vi "Check Writer Backpressure.vi"(8 "error in (no error)":errorcluster, 10 "Timeout (ms)":i32, 11 "CIF_CIPC_Chn in":refnum<class "CIF_CIPC_Chn.lvclass">) -> (0 "error out":errorcluster, 2 "timed out?":bool)   [LabVIEW 2021, in "CIF_CIPC_Chn.lvclass"]
uses:
  CIF_CIPC_Chn.lvclass
  D:/dev/Packages/CIF_Channels_Core/src/CIFChannels/CIFChannels.lvclass
  CIFChannels/CIFChannels.lvclass/CIFChannels.ctl
  CIF_CIPC_Chn.lvclass/CIF_CIPC_Chn.ctl
  CIFChannels/Accessors/Read FIFO Backpressure.vi
  080cd5e1-c136-44b9-98fd-184f8e575b7e.vi/3d5c1244-b460-4622-96d1-ee1e369932ac.vi
  <vilib>/CIF Foundation/CIF CIPC/Utilities/Get Size.vi
  080cd5e1-c136-44b9-98fd-184f8e575b7e.vi/b3361ac9-0b85-4d75-8feb-76d028d0c03f.vi
  <vilib>/CIF Foundation/CIF CIPC/SubVIs/Get Element Write Position.vi
  <vilib>/CIF Foundation/CIF CIPC/SubVIs/Wait For N Elements Available.vi
  <vilib>/CIF Foundation/CIF CIPC/SubVIs/Check Error.vi
  <vilib>/CIF Foundation/CIF CIPC/SubVIs/Get dll Path.vi
  <vilib>/CIF Foundation/CIF CIPC/SubVIs/Get Element Read Position.vi
  <vilib>/CIF Foundation/CIF CIPC/SubVIs/Set Element Read Position.vi
  <vilib>/Utility/error.llb/Trim Whitespace.vi
  <vilib>/Utility/error.llb/Error Cluster From Error Code.vi
  <vilib>/CIF Foundation/CIF CIPC/SubVIs/Get Element Info Variant.vi
  7796537b-0e69-421b-96bb-30a861203fb6.vi
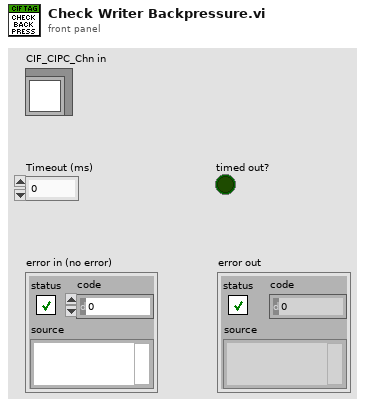
[diagram p1: front panel]
types:
  T1 = typedef "CIF_CIPC_Chn.lvclass/Buffer Configuration Data.ctl" = cluster{"Total Size":u32, "Read Size":u32, "Read Offset":u32, "CIPC BP References":T2, "Override CIPC Name":string, "Encoder Data":string}
  T2 = typedef "CIF_NI_CIPC.lvlib/Backpressure References.ctl" = cluster{"CIPC Reference":u64, "CIPC BP Reference":u64}
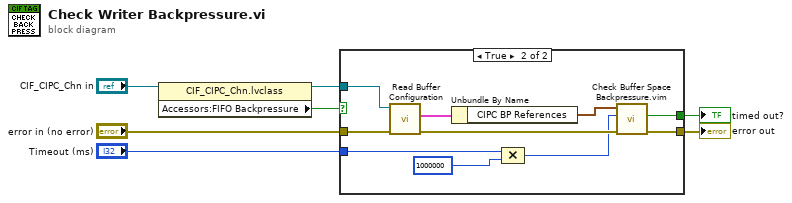
[diagram p0: block diagram]
diagram:
  n1 = property class="CIF_CIPC_Chn.lvclass"(reference="CIF_CIPC_Chn in") -> (reference out=w6:refnum<class "CIF_CIPC_Chn.lvclass">, "Accessors:FIFO Backpressure"=w7:bool)  [unwired: 1 in, 1 out]
  n2 = case shown="True" w7 {
    tunnel: [w8 w9] -> w2
    tunnel: "error in (no error)" -> [w8 w17]
    tunnel: w6 -> [_ w18]
    tunnel: [_ w13] -> w1
    tunnel: "Timeout (ms)" -> [_ w12]
    frame False {
    }
    frame True {
      n3 = call "Read Buffer Configuration.vi"("error in (no error)"=w17, "CIF_CIPC_Chn in"=w18) -> ("error out"=w14:errorcluster, "Buffer Configuration"=w16:T1)  [unwired: 7 in, 1 out]
      n4 = Unbundle By Name(w16) -> ("CIPC BP References"=w15:T2)
      n5 = Compound Arithmetic op=MULTIPLY(w12, 1000000 ("value")) -> (w10:i32)
      n6 = call "Check Buffer Space Backpressure.vim"("error in (no error)"=w14, "Timeout (ns)"=w10, "CIPC BP References in"=w15) -> ("error out"=w9:errorcluster, "Timeout"=w13:bool)  [unwired: 6 in, 1 out]
    }
  }
  "error out" <- w2
  "timed out?" <- w1
